vi "Servo update actual position.vi"(8 "error in (no error)":errorcluster, 11 "Status in":T1) -> (0 "error out":errorcluster, 3 "Status out":T1)   [LabVIEW 2017]
doc: "Read actual position and check if target is reached.\nIn case of reading error it returns that is out of target, in positive infinity position, and disconnected."
uses:
  ctl/Servo state.ctl
  ctl/Servo variables.ctl
  ctl/Servo constants.ctl
  ctl/Axis names.ctl
  <vilib>/addons/eal4LabVIEW/eal4LabVIEW.lvlib
  Servo drive module.lvlib
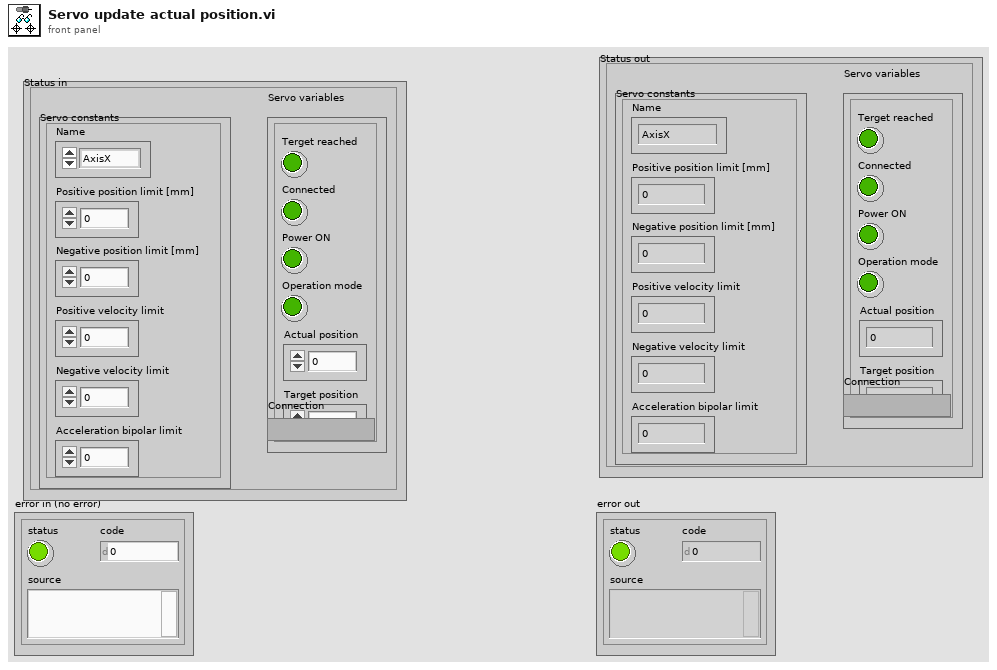
[diagram p1: front panel]
types:
  T1 = typedef "Servo drive module.lvlib/Servo state.ctl" = cluster{"Servo variables":T2, "Servo constants":T3, "Connection":variant}
  T2 = typedef "Servo drive module.lvlib/Servo variables.ctl" = cluster{"Terget reached":bool, "Connected":bool, "Power ON":bool, "Operation mode":bool, "Actual position":dbl, "Target position":dbl}
  T3 = typedef "Servo drive module.lvlib/Servo constants.ctl" = cluster{"Name":T4, "Positive position limit [mm]":dbl, "Negative position limit [mm]":dbl, "Positive velocity limit":dbl, "Negative velocity limit":dbl, "Acceleration bipolar limit":dbl}
  T4 = typedef "Servo drive module.lvlib/Axis names.ctl" = enum16{"AxisX", "AxisY", "AxisZ_left", "AxisZ_middle", "AxisZ_right"}
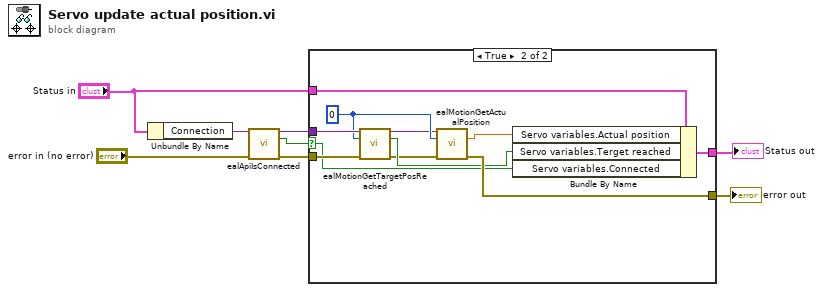
[diagram p0: block diagram]
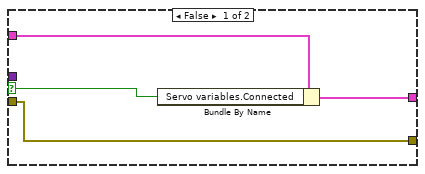
[diagram p2: hidden frame]
diagram:
  n1 = Unbundle By Name("Status in") -> ("Connection"=w5:variant)
  n2 = call <vilib>:"ealApiIsConnected.vi"("connection in"=w5, "error in (no error)"="error in (no error)") -> ("connection out"=w4:variant, "is connected"=w1:bool, "error out"=w2:errorcluster)  [unwired: 11 in]
  n3 = case shown="True" w1 {
    selector: w1 -> [w11 w13]
    tunnel: [w9 w23] -> w8
    tunnel: [w10 w22] -> w7
    tunnel: "Status in" -> [w12 w20]
    tunnel: w4 -> [_ w19]
    tunnel: w2 -> [w9 w18]
    frame False {
      n4 = Bundle By Name(cluster=w12, "Servo variables.Connected"=w11) -> (w10:T1)
    }
    frame True {
      w16 = 0
      n5 = call <vilib>:"ealMotionGetTargetPosReached.vi"("connection in"=w19, "slave index"=w16, "error in (no error)"=w18) -> ("connection out"=w15:variant, "target position reached"=w17:bool, "error out"=w14:errorcluster)  [unwired: 10 in]
      n6 = call <vilib>:"ealMotionGetActualPosition.vi"("connection in"=w15, "slave index"=w16, "error in (no error)"=w14) -> ("getActualPosition"=w21:dbl, "error out"=w23:errorcluster)  [unwired: 10 in, 1 out]
      n7 = Bundle By Name(cluster=w20, "Servo variables.Actual position"=w21, "Servo variables.Terget reached"=w17, "Servo variables.Connected"=w13) -> (w22:T1)
    }
  }
  "error out" <- w8
  "Status out" <- w7
